vi "KE622x -- 2182 -A Set Digital Filter Window.vi"(0 "622x Resource In":refnum<visa-resource-name>, 1 "Check For SCPI Errors? (T)":bool=TRUE, 7 "Filter Window In (%)":T1=0.01 min=0.0 max=10.0 step=0.01 format="%.2f", 11 "error in (no error)":errorcluster, 12 "Read Back Set Value? (T)":bool=TRUE) -> (4 "622x Resource Out (dupl)":refnum<visa-resource-name>, 15 "error out":errorcluster)   [LabVIEW 2019, in "Keithley 622x.lvlib"]
uses:
  Keithley 622x.lvlib
  Typedefs/KE2182 -- Filter Window.ctl
panel:
  out "Filter Window Out (%)":T1=0.01 min=0.0 max=10.0 step=0.01 format="%.2f"
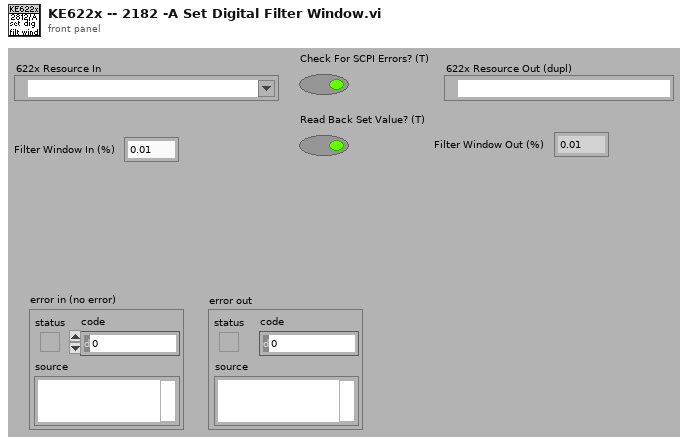
[diagram p1: front panel]
types:
  T1 = typedef "Keithley 622x.lvlib/KE2182 -- Filter Window.ctl" = dbl
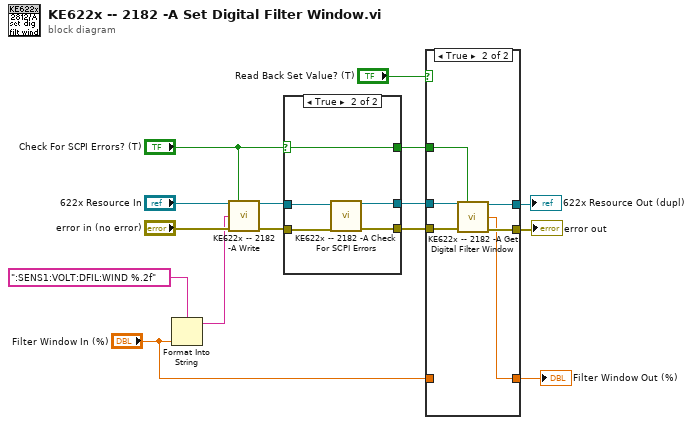
[diagram p0: block diagram]
diagram:
  n1 = Format Into String(format string=":SENS1:VOLT:DFIL:WIND %.2f", "Filter Window In (%)") -> (resulting string=w10:string)  [unwired: 2 in, 1 out]
  n2 = call "KE622x -- 2182 -A Write.vi"("Resource In"="622x Resource In", "Check For SCPI Errors? (T)"="Check For SCPI Errors? (T)", "2182-A Write String"=w10, "error in (no error)"="error in (no error)") -> ("Resource Out (dupl)"=w13:refnum<visa-resource-name>, "error out"=w9:errorcluster)  [unwired: 10 in]
  n3 = case shown="True" "Check For SCPI Errors? (T)" {
    selector: "Check For SCPI Errors? (T)" -> [w16 w19]
    tunnel: w13 -> [w18 w23]
    tunnel: w9 -> [w17 w22]
    tunnel: [w18 w21] -> w8
    tunnel: [w17 w20] -> w7
    tunnel: [w16 w19] -> w6
    frame False {
    }
    frame True {
      n4 = call "KE622x -- 2182 -A Check For SCPI Errors.vi"("VISA Resource In"=w23, "error in (no error)"=w22) -> ("VISA Resource Out (dupl)"=w21:refnum<visa-resource-name>, "error out"=w20:errorcluster)  [unwired: 10 in, 2 out]
    }
  }
  n5 = case shown="True" "Read Back Set Value? (T)" {
    tunnel: w8 -> [w25 w32]
    tunnel: w7 -> [w24 w31]
    tunnel: w6 -> [_ w30]
    tunnel: [w25 w29] -> w5
    tunnel: [w24 w28] -> w4
    tunnel: "Filter Window In (%)" -> [w26 _]
    tunnel: [w26 w27] -> w1
    frame False {
    }
    frame True {
      n6 = call "KE622x -- 2182 -A Get Digital Filter Window.vi"("622x Resource In"=w32, "Check For SCPI Errors? (T)"=w30, "error in (no error)"=w31) -> ("622x Resource Out (dupl)"=w29:refnum<visa-resource-name>, "Filter Window (%)"=w27:T1, "error out"=w28:errorcluster)  [unwired: 10 in]
    }
  }
  "622x Resource Out (dupl)" <- w5
  "error out" <- w4
  "Filter Window Out (%)" <- w1
